vi "Set Video Mode.vi"(8 "error in (no error)":errorcluster, 9 "Video Line Marker (1)":i32=1, 10 "Video Format (0: NTSC)":u32(ring) items=["NTSC", "PAL", "PALM (for PAL-M)", "SECAM"], 11 "VISA resource name":refnum<visa-resource-name>) -> (0 "error out":errorcluster, 3 "VISA resource name out":refnum<visa-resource-name>)   [LabVIEW 2011, in "Fluke 5XXX Series Multicalibrators.lvlib"]
doc: "This VI selects the format for Video scope mode and programs the Video mode line marker location.\n\nNote:\n\nThis VI is available only for instrument models 5500A and 5520A with oscilloscope option SC600 (SC1100)."
uses:
  Fluke 5XXX Series Multicalibrators.lvlib
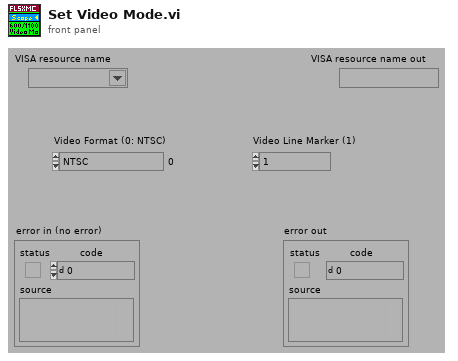
[diagram p1: front panel]
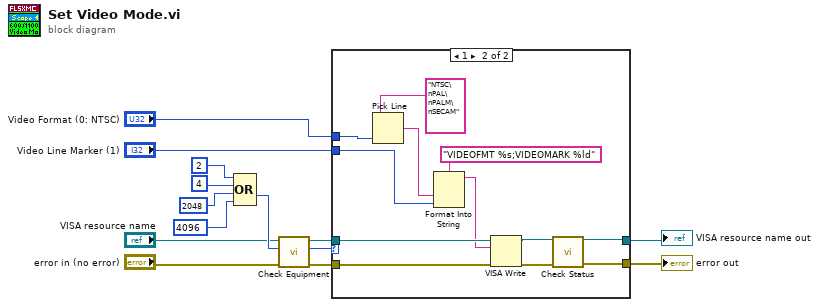
[diagram p0: block diagram]
diagram:
  n1 = Compound Arithmetic op=OR(2 ("Numeric"), 4 ("Numeric"), 2048 ("Numeric"), 4096 ("Numeric")) -> (w8:i32)
  n2 = call "Check Equipment.vi"("error in (no error)"="error in (no error)", "Bit Mask"=w8, "VISA resource name"="VISA resource name") -> ("error out"=w11:errorcluster, "Present?"=w10:u32, "VISA resource name out"=w9:refnum<visa-resource-name>)  [unwired: 6 in]
  n3 = case shown="1" w10 {
    tunnel: [w15 w22] -> w3
    tunnel: w11 -> [w16 w27]
    tunnel: w9 -> [w15 w26]
    tunnel: [w16 w25] -> w4
    tunnel: "Video Line Marker (1)" -> [_ w18]
    tunnel: "Video Format (0: NTSC)" -> [_ w17]
    frame 0, Default {
    }
    frame 1 {
      n4 = Pick Line(multi-line string="NTSC\nPAL\nPALM\nSECAM", line index=w17) -> (output string=w21:string)  [unwired: 1 in]
      n5 = Format Into String(format string="VIDEOFMT %s;VIDEOMARK %ld" ("Reset Command"), w21, w18) -> (resulting string=w19:string)  [unwired: 2 in, 1 out]
      n6 = VISA Write(VISA resource name=w26, write buffer=w19, error in (no error)=w27) -> (VISA resource name out=w23:refnum<visa-resource-name>, error out=w24:errorcluster)  [unwired: 1 out]
      n7 = call "Check Status.vi"("VISA resource name"=w23, "error in (no error)"=w24) -> ("VISA resource name out"=w22:refnum<visa-resource-name>, "error out"=w25:errorcluster)  [unwired: 12 in]
    }
  }
  "VISA resource name out" <- w3
  "error out" <- w4
